vi "SetUp_Action.vi"(8 "error in":errorcluster caption="错误输入", 11 "GuiRef":T1) -> (0 "error out":errorcluster caption="错误输出", 3 "ScanSNOK":bool)   [LabVIEW 2013]
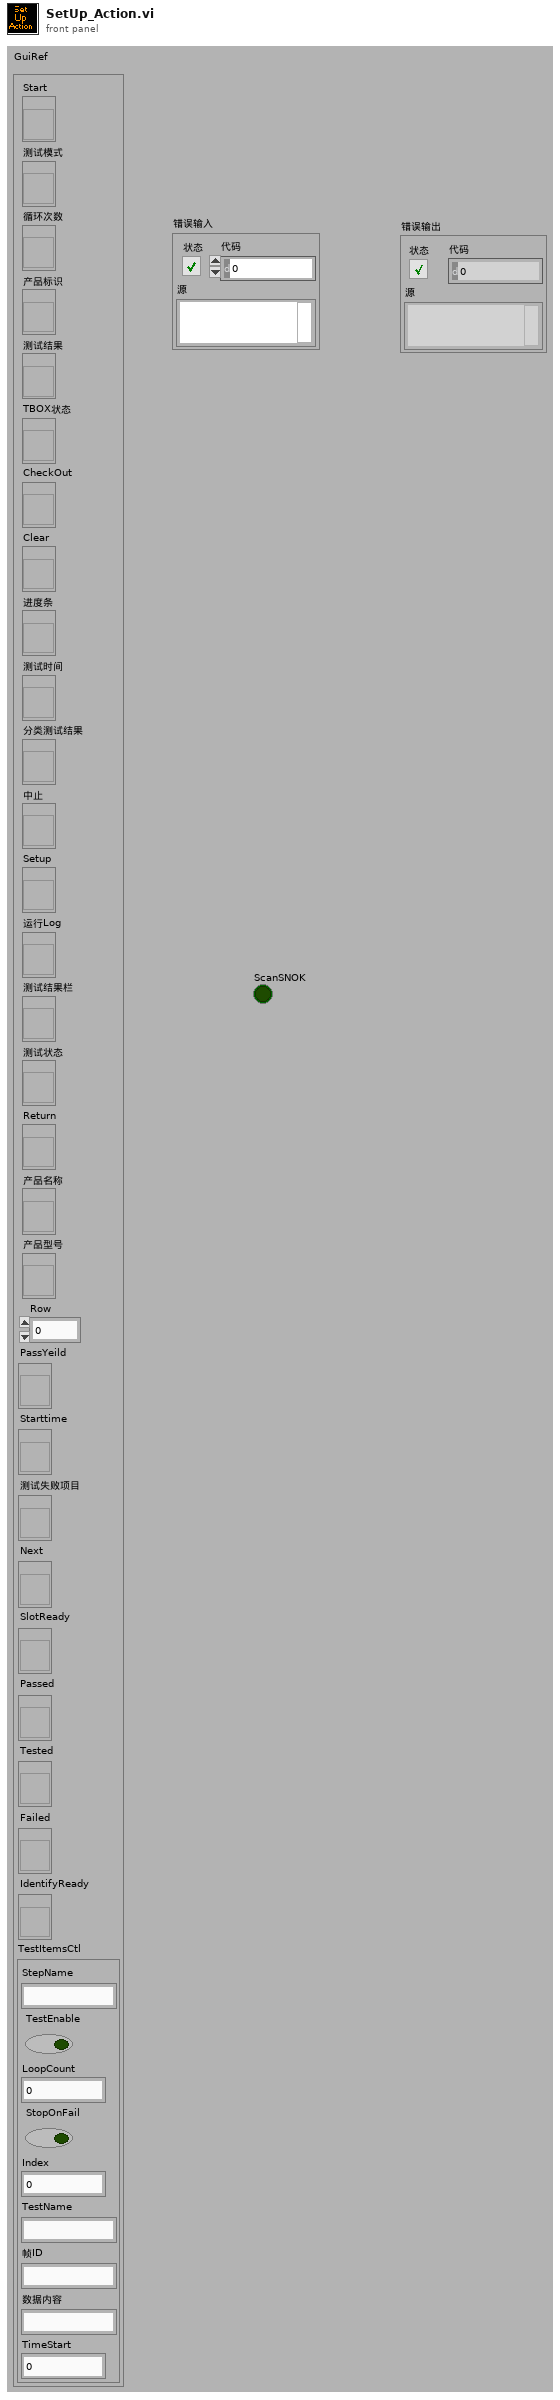
[diagram p1: front panel]
types:
  T1 = typedef "控件.ctl" = cluster{"Start":refnum<vi>, "测试模式":refnum<vi>, "循环次数":refnum<vi>, "产品标识":refnum<vi>, "测试结果":refnum<vi>, "TBOX状态":refnum<vi>, "CheckOut":refnum<vi>, "Clear":refnum<vi>, "进度条":refnum<vi>, "测试时间":refnum<vi>, "分类测试结果":refnum<vi>, "中止":refnum<vi>, "Setup":refnum<vi>, "运行Log":refnum<vi>, "测试结果栏":refnum<vi>, "测试状态":refnum<vi>, "Return":refnum<vi>, "产品名称":refnum<vi>, "产品型号":refnum<vi>, "Row":i32, "PassYeild":refnum<vi>, "Starttime":refnum<vi>, "测试失败项目":refnum<vi>, "Next":refnum<vi>, "SlotReady":refnum<vi>, "Passed":refnum<vi>, "Tested":refnum<vi>, "Failed":refnum<vi>, "IdentifyReady":refnum<vi>, "TestItemsCtl":cluster{"StepName":string, "TestEnable":bool, "LoopCount":u32, "StopOnFail":bool, "Index":u32, "TestName":string, "帧ID":string, "数据内容":string, "TimeStart":u32}}
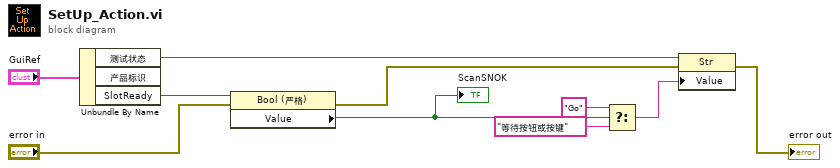
[diagram p0: block diagram]
diagram:
  n1 = Unbundle By Name("GuiRef") -> ("测试状态"=w8:refnum<vi>, "SlotReady"=w9:refnum<vi>)  [unwired: 1 out]
  n2 = property class="Bool (严格)"(reference=w9, error in="error in") -> (error out=w2:errorcluster, "Value"=w7:bool)  [unwired: 1 out]
  "ScanSNOK" <- w7
  n3 = Select(t="Go", s=w7, f="等待按钮或按键") -> (s? t:f=w4:string)
  n4 = property class="Str"(reference=w8, error in=w2, "Value"=w4) -> (error out=→"error out":errorcluster)  [unwired: 1 out]
